vi "GetDependentInfo.vi"(7 "Project ref":refnum<vi>, 8 "error in (no error)":errorcluster, 11 "ProjectItem in":refnum<class "ProjectItem.lvclass">) -> (0 "error out":errorcluster, 1 "Dependent owning libs":string[](array[string]), 2 "Dependent paths":path[](array[path]), 3 "ProjectItem out":refnum<class "ProjectItem.lvclass">)   [LabVIEW 2019, in "SolutionBuilder.lvlib" / "ProjectItem.lvclass"]
uses:
  ProjectItem.lvclass
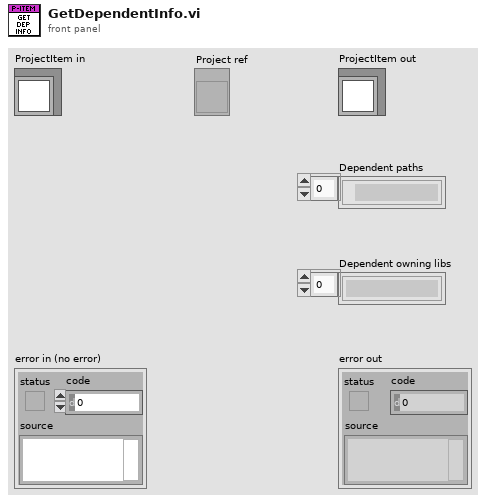
[diagram p1: front panel]
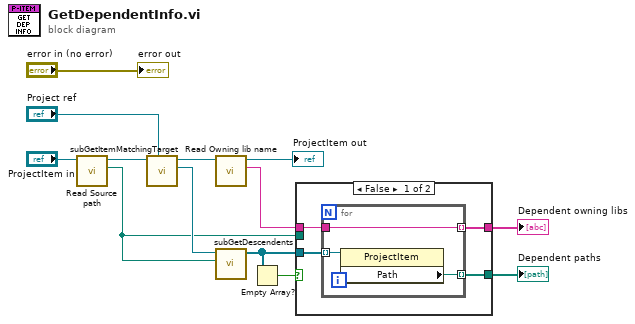
[diagram p0: block diagram]
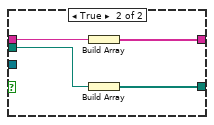
[diagram p2: hidden frame]
diagram:
  n1 = call-dynamic "Read Source path.vi"("ProjectItem in"="ProjectItem in") -> ("Source path"=w9:path, "ProjectItem out"=w11:refnum<class "ProjectItem.lvclass">)  [unwired: 9 in]
  n2 = call "subGetItemMatchingTarget.vi"("Project ref"="Project ref", "ProjectItem in"=w11) -> ("TargetItem Ref"=w12:refnum<vi>, "ProjectItem out"=w7:refnum<class "ProjectItem.lvclass">)  [unwired: 7 in, 1 out]
  n3 = call-dynamic "Read Owning lib name.vi"("ProjectItem in"=w7) -> ("Owning lib name"=w6:string, "ProjectItem out"=→"ProjectItem out":refnum<class "ProjectItem.lvclass">)  [unwired: 9 in]
  n4 = call "subGetDescendents.vi"("Source path"=w9, "TargetItem in"=w12) -> ("Get All Descendents"=w10:refnum<vi>[])  [unwired: 9 in]
  n5 = Empty Array?(array=w10) -> (empty?=w8:bool)
  n6 = case shown="False" w8 {
    tunnel: w10 -> [w17 _]
    tunnel: w9 -> [_ w24]
    tunnel: w6 -> [w16 w22]
    tunnel: [w15 w21] -> w3
    tunnel: [w14 w23] -> w2
    frame False {
      n7 = for {
        tunnel: w17 -> [w20] mode=indexing
        tunnel: [w19] -> w14 mode=indexing
        tunnel: w16 -> [w18]
        tunnel: [w18] -> w15 mode=indexing
        n8 = property class="ProjectItem"(reference=w20) -> ("Path"=w19:path)  [unwired: 1 in, 2 out]
      }
    }
    frame True {
      n9 = Build Array(w22) -> (w21:string[])
      n10 = Build Array(w24) -> (w23:path[])
    }
  }
  "Dependent owning libs" <- w3
  "Dependent paths" <- w2
  "error out" <- "error in (no error)"
